vi "Sequence.Preview.vi"(8 "error in (no error)":errorcluster, 11 "State Variables":T1) -> (0 "error out":errorcluster)   [LabVIEW 2013, in "Simple Sequence Editor.lvlib"]
uses:
  Simple Sequence Editor.lvlib
  Types/StateVariables.ctl
  Types/ChannelProperties.ctl
panel:
  out "Graph":waveform(dbl)[](graph)
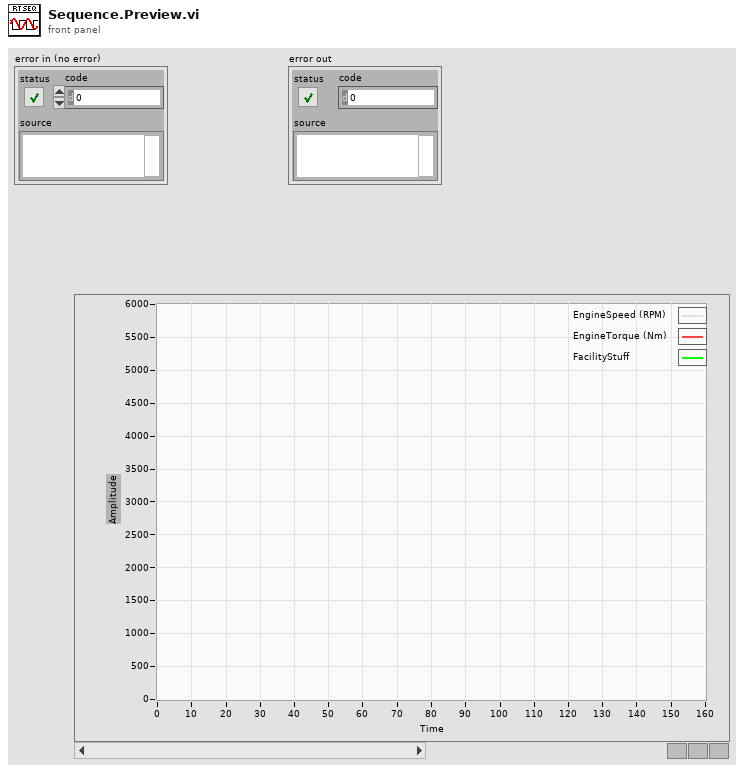
[diagram p1: front panel]
types:
  T1 = typedef "Simple Sequence Editor.lvlib/StateVariables.ctl" = cluster{"Aliases.All":T2[], "Aliases.Outputs":T2[], "UI.Sequence#ofColumns":i32, "SysDef.Path":path, "UI.SequenceRef":refnum<vi>, "UI.StepInformationRef":refnum<vi>, "UI.AbortRef":refnum<vi>, "UI.GraphRef":refnum<vi>, "UI.ViewRef":refnum<vi>, "UI.IterationsRef":refnum<vi>, "UI.IterationInformationRef":refnum<vi>}
  T2 = typedef "Simple Sequence Editor.lvlib/ChannelProperties.ctl" = cluster{"Name":string, "NodePath":string, "ScaleUnits":string}
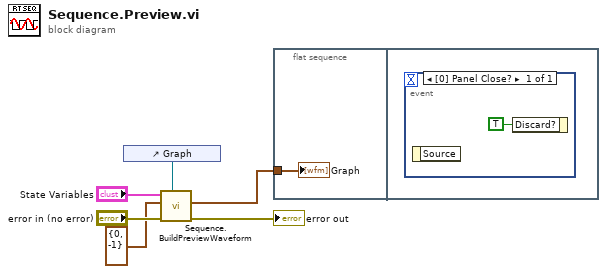
[diagram p0: block diagram]
diagram:
  n1 = control-ref of="Graph"() -> (w3:refnum<vi>)
  n2 = call "Sequence.BuildPreviewWaveform.vi"("WaveformGraph in"=w3, "error in (no error)"="error in (no error)", "Rows"=cluster{"Start Index":i32, "Length":i32} {"Start Index"=0, "Length"=-1}, "input cluster"="State Variables") -> ("error out"=→"error out":errorcluster, "Wavefrom"=w4:waveform(dbl)[])  [unwired: 5 in, 1 out]
  n3 = flat-sequence {
    tunnel: w4 -> [w7]
    frame #0 {
      "Graph" <- w7
    }
    frame #1 {
      n4 = event shown="[0] Panel Close?" {
        selector: _ -> [_]
        dyn-events: _ -> [_]
        timeout: _ -> [_]
        event Panel Close? {
          n5 = event-data() -> ()  [unwired: 1 in, 1 out]
          n6 = event-data("Discard?"=TRUE) -> ()  [unwired: 1 in, 1 out]
        }
      }
    }
  }
